vi "HCalGlove.vi"(4 "error in (no error)":errorcluster, 5 "RH?":bool, 7 "VISA Resource In":refnum<visa-resource-name>) -> (0 "error out":errorcluster, 2 "Calibration Array":u8[][](array[numeric]), 3 "VISA Resource Out":refnum<visa-resource-name>)   [LabVIEW 2009]
uses:
  HCalGet.vi
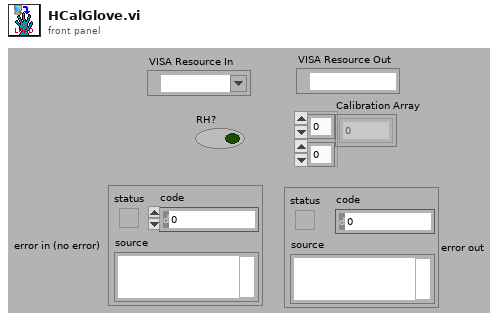
[diagram p1: front panel]
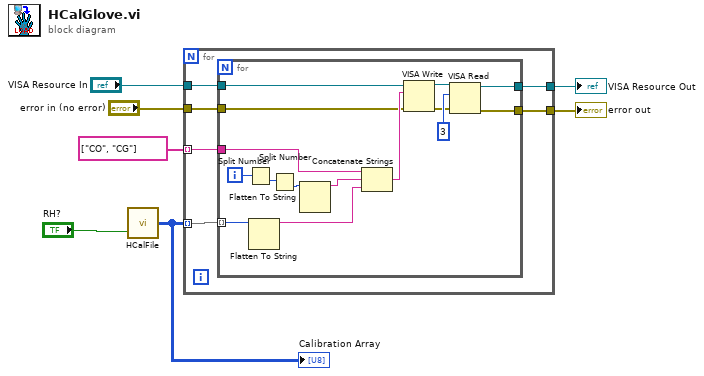
[diagram p0: block diagram]
diagram:
  n1 = call-poly "HCalFile.vi"("RH?"="RH?") -> ("Calibration Array"=w6:u8[][])  [unwired: 1 in]
  "Calibration Array" <- w6
  n2 = for {
    tunnel: w6 -> [w13] mode=indexing
    tunnel: string[] ["CO", "CG"] -> [w12] mode=indexing
    tunnel: "VISA Resource In" -> [w11]
    tunnel: "error in (no error)" -> [w10]
    tunnel: [w9] -> w2
    tunnel: [w8] -> w1
    n3 = for {
      tunnel: w13 -> [w28] mode=indexing
      tunnel: w12 -> [w24]
      tunnel: w11 -> [w20]
      tunnel: w10 -> [w16]
      tunnel: [w15] -> w9
      tunnel: [w14] -> w8
      i -> [w27]
      n4 = Split Number(x=w27) -> (lo(x)=w26:u16)  [unwired: 1 out]
      n5 = Flatten To String(anything=w28) -> (data string=w22:string)  [unwired: 3 in, 2 out]
      n6 = Split Number(x=w26) -> (lo(x)=w25:u8)  [unwired: 1 out]
      n7 = Flatten To String(anything=w25) -> (data string=w23:string)  [unwired: 3 in, 2 out]
      n8 = Concatenate Strings(w24, w23, w22) -> (w21:string)
      n9 = VISA Write(VISA resource name=w20, write buffer=w21, error in (no error)=w16) -> (VISA resource name out=w18:refnum<visa-resource-name>, error out=w17:errorcluster)  [unwired: 1 out]
      n10 = VISA Read(VISA resource name=w18, byte count=u32 3, error in (no error)=w17) -> (VISA resource name out=w14:refnum<visa-resource-name>, error out=w15:errorcluster)  [unwired: 2 out]
    }
  }
  "error out" <- w2
  "VISA Resource Out" <- w1
